vi "BP_Load Sound.vi"() -> (0 "error out":errorcluster, 2 "Sound Array":T1[](array[typedef]) format="%.0x", 3 "task ID out":T1 format="%.0x")   [LabVIEW 2019]
uses:
  <vilib>/sound2/lvsound2.llb/Sound Output Task ID.ctl
panel:
  in  "Sound files":string[](array[string])=["1800 warning.wav", "1500 warning.wav", "200 warning.wav"]
  out "appended path":path
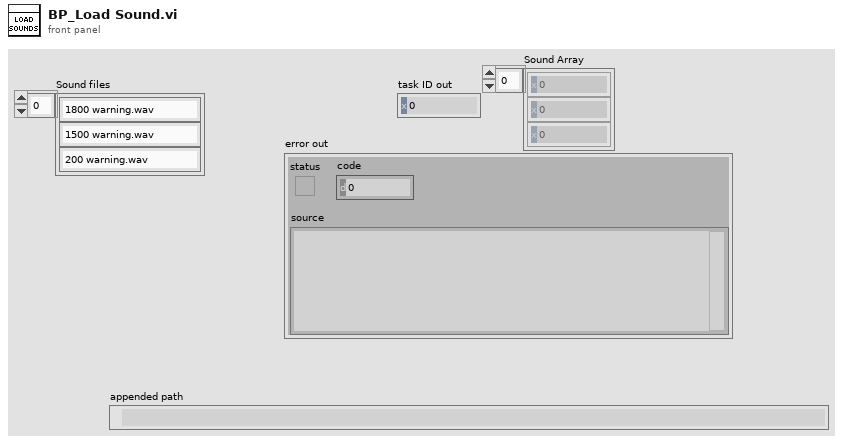
[diagram p1: front panel]
types:
  T1 = typedef "Sound Output Task ID.ctl" = u32
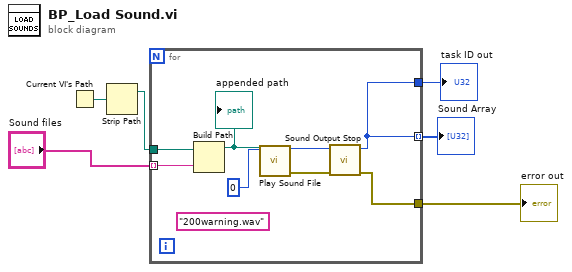
[diagram p0: block diagram]
diagram:
  n1 = Current VI's Path() -> (path=w6:path)
  n2 = Strip Path(path=w6) -> (stripped path=w4:path)  [unwired: 1 out]
  n3 = for {
    tunnel: [w14] -> w5
    tunnel: w4 -> [w13]
    tunnel: [w7] -> w3
    tunnel: "Sound files" -> [w8] mode=indexing
    tunnel: [w7] -> w2 mode=indexing
    (unwired) "200warning.wav" ("name or relative path")
    n4 = Build Path(base path=w13, name or relative path=w8) -> (appended path=w12:path)
    "appended path" <- w12
    n5 = call <vilib>:"Play Sound File.vi"("path"=w12, "device ID"=u32 0) -> ("error out"=w11:errorcluster, "task ID"=w10:T1)  [unwired: 8 in]
    n6 = call <vilib>:"Sound Output Stop.vi"("error in (no error)"=w11, "task ID"=w10) -> ("error out"=w14:errorcluster, "task ID out"=w7:T1)  [unwired: 8 in]
  }
  "error out" <- w5
  "task ID out" <- w3
  "Sound Array" <- w2
